vi "startSweep.vi"(8 "error in (no error)":errorcluster, 11 "Instrument.LockinAPI in":refnum<class "Instrument.LockinAPI.lvclass">) -> (0 "error out":errorcluster, 3 "Instrument.LockinAPI out":refnum<class "Instrument.LockinAPI.lvclass">)   [LabVIEW 2019, in "Instrument.LockinAPI.lvclass"]
doc: "API to assert the trigger.\n\nIf address=\"\", this API reads from localhost\nIf address is remote lockin, you need to add this computer to allowed whitelist on the lockin computer you are trying to access."
uses:
  Instrument.LockinAPI.lvclass
  Typedefs/LockinAPI.setState.states--Enum.ctl
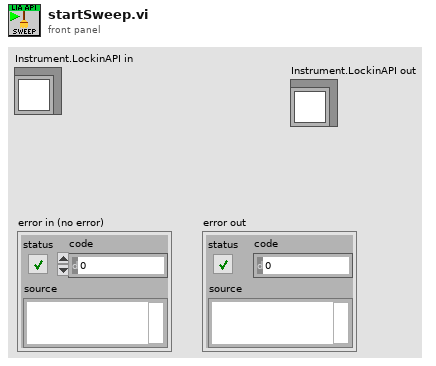
[diagram p1: front panel]
types:
  T1 = typedef "Instrument.LockinAPI.lvclass/LockinAPI.setState.states--Enum.ctl" = enum16{"start", "stop", "reset", "start sweep", "stop sweep"}
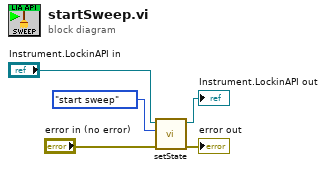
[diagram p0: block diagram]
diagram:
  n1 = call-dynamic "setState.vi"("error in (no error)"="error in (no error)", "state"=LockinAPI.setState.states--Enum."start sweep" ("setState state"), "Instrument.LockinAPI in"="Instrument.LockinAPI in") -> ("error out"=→"error out":errorcluster, "Instrument.LockinAPI out"=→"Instrument.LockinAPI out":refnum<class "Instrument.LockinAPI.lvclass">)  [unwired: 7 in]
